vi "Bila-Sonatina.vi"(11 "NXT/EV3":T1) -> (3 "NXT/EV3 2":T1)   [LabVIEW 2016]
uses:
  <vilib>/NXT/Subs/LVHSConnector.ctl
  <vilib>/NXT/LegoClasses/BrickReference/BrickReference.lvclass
  <vilib>/NXT/Dual Mode Library/Display/drawText_Center.vi
  <vilib>/NXT/Dual Mode Library/Sound/PlayG.vi
  <vilib>/NXT/Dual Mode Library/Waits/Wait_Num.vi
  <vilib>/NXT/Dual Mode Library/Sound/PlayB.vi
  <vilib>/NXT/Dual Mode Library/Sound/PlayA.vi
  <vilib>/NXT/Dual Mode Library/Sound/PlayD.vi
  <vilib>/NXT/Dual Mode Library/Sound/PlayC.vi
  <vilib>/NXT/Dual Mode Library/Sound/PlayE.vi
  <vilib>/NXT/Dual Mode Library/Sound/PlayFsharp.vi
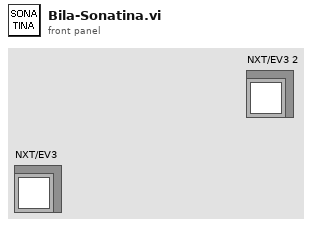
[diagram p1: front panel]
types:
  T1 = typedef "LVHSConnector.ctl" = refnum<class "BrickReference.lvclass">
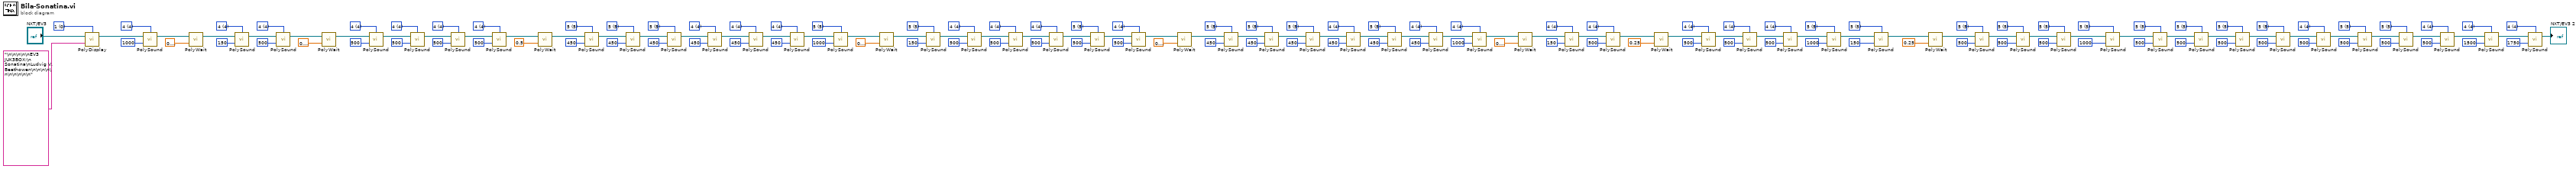
[diagram p0: block diagram]
diagram:
  w6 = u16 4 items=["3"=3, "4"=4, "5"=5, "6"=6, "7"=7] ("Octave")
  w10 = u16 5 items=["3"=3, "4"=4, "5"=5, "6"=6, "7"=7] ("Octave")
  w17 = u16 4 items=["3"=3, "4"=4, "5"=5, "6"=6, "7"=7] ("Octave")
  w20 = u16 4 items=["3"=3, "4"=4, "5"=5, "6"=6, "7"=7] ("Octave")
  w21 = u16 5 items=["3"=3, "4"=4, "5"=5, "6"=6, "7"=7] ("Octave")
  w24 = u16 4 items=["3"=3, "4"=4, "5"=5, "6"=6, "7"=7] ("Octave")
  w25 = u16 5 items=["3"=3, "4"=4, "5"=5, "6"=6, "7"=7] ("Octave")
  w28 = u16 5 items=["3"=3, "4"=4, "5"=5, "6"=6, "7"=7] ("Octave")
  w29 = u16 5 items=["3"=3, "4"=4, "5"=5, "6"=6, "7"=7] ("Octave")
  w32 = u16 5 items=["3"=3, "4"=4, "5"=5, "6"=6, "7"=7] ("Octave")
  w42 = u16 5 items=["3"=3, "4"=4, "5"=5, "6"=6, "7"=7] ("Octave")
  w41 = u16 5 items=["3"=3, "4"=4, "5"=5, "6"=6, "7"=7] ("Octave")
  w38 = u16 5 items=["3"=3, "4"=4, "5"=5, "6"=6, "7"=7] ("Octave")
  w37 = u16 5 items=["3"=3, "4"=4, "5"=5, "6"=6, "7"=7] ("Octave")
  w34 = u16 5 items=["3"=3, "4"=4, "5"=5, "6"=6, "7"=7] ("Octave")
  w62 = u16 5 items=["3"=3, "4"=4, "5"=5, "6"=6, "7"=7] ("Octave")
  w63 = u16 4 items=["3"=3, "4"=4, "5"=5, "6"=6, "7"=7] ("Octave")
  w66 = u16 4 items=["3"=3, "4"=4, "5"=5, "6"=6, "7"=7] ("Octave")
  w67 = u16 4 items=["3"=3, "4"=4, "5"=5, "6"=6, "7"=7] ("Octave")
  w70 = u16 4 items=["3"=3, "4"=4, "5"=5, "6"=6, "7"=7] ("Octave")
  w71 = u16 4 items=["3"=3, "4"=4, "5"=5, "6"=6, "7"=7] ("Octave")
  w74 = u16 4 items=["3"=3, "4"=4, "5"=5, "6"=6, "7"=7] ("Octave")
  w84 = u16 4 items=["3"=3, "4"=4, "5"=5, "6"=6, "7"=7] ("Octave")
  w85 = u16 5 items=["3"=3, "4"=4, "5"=5, "6"=6, "7"=7] ("Octave")
  w87 = u16 4 items=["3"=3, "4"=4, "5"=5, "6"=6, "7"=7] ("Octave")
  w90 = u16 5 items=["3"=3, "4"=4, "5"=5, "6"=6, "7"=7] ("Octave")
  w91 = u16 5 items=["3"=3, "4"=4, "5"=5, "6"=6, "7"=7] ("Octave")
  w94 = u16 5 items=["3"=3, "4"=4, "5"=5, "6"=6, "7"=7] ("Octave")
  w96 = u16 4 items=["3"=3, "4"=4, "5"=5, "6"=6, "7"=7] ("Octave")
  w111 = u16 5 items=["3"=3, "4"=4, "5"=5, "6"=6, "7"=7] ("Octave")
  w108 = u16 4 items=["3"=3, "4"=4, "5"=5, "6"=6, "7"=7] ("Octave")
  w107 = u16 4 items=["3"=3, "4"=4, "5"=5, "6"=6, "7"=7] ("Octave")
  w104 = u16 4 items=["3"=3, "4"=4, "5"=5, "6"=6, "7"=7] ("Octave")
  w103 = u16 5 items=["3"=3, "4"=4, "5"=5, "6"=6, "7"=7] ("Octave")
  w100 = u16 5 items=["3"=3, "4"=4, "5"=5, "6"=6, "7"=7] ("Octave")
  w124 = u16 4 items=["3"=3, "4"=4, "5"=5, "6"=6, "7"=7] ("Octave")
  w127 = u16 4 items=["3"=3, "4"=4, "5"=5, "6"=6, "7"=7] ("Octave")
  w131 = u16 4 items=["3"=3, "4"=4, "5"=5, "6"=6, "7"=7] ("Octave")
  w128 = u16 5 items=["3"=3, "4"=4, "5"=5, "6"=6, "7"=7] ("Octave")
  w134 = u16 5 items=["3"=3, "4"=4, "5"=5, "6"=6, "7"=7] ("Octave")
  w137 = u16 5 items=["3"=3, "4"=4, "5"=5, "6"=6, "7"=7] ("Octave")
  w150 = u16 4 items=["3"=3, "4"=4, "5"=5, "6"=6, "7"=7] ("Octave")
  w151 = u16 4 items=["3"=3, "4"=4, "5"=5, "6"=6, "7"=7] ("Octave")
  w154 = u16 4 items=["3"=3, "4"=4, "5"=5, "6"=6, "7"=7] ("Octave")
  w155 = u16 4 items=["3"=3, "4"=4, "5"=5, "6"=6, "7"=7] ("Octave")
  w158 = u16 4 items=["3"=3, "4"=4, "5"=5, "6"=6, "7"=7] ("Octave")
  w159 = u16 4 items=["3"=3, "4"=4, "5"=5, "6"=6, "7"=7] ("Octave")
  w162 = u16 4 items=["3"=3, "4"=4, "5"=5, "6"=6, "7"=7] ("Octave")
  w164 = i16 0 items=["1", "2", "3", "4", "5", "6", "7", "8", "9", "10", "11", "12"] ("Line")
  n1 = call-poly <vilib>:"PolyDisplay.vi"("Text"="\n\n\n\n\nEV3 JUK3BOX:\n Sonatina\nLudvig V. Beethowen\n\n\n\n\n\n\n\n\n\n", "NXT/EV3"="NXT/EV3", "Line"=w164) -> ("NXT/EV3"=w144:T1)  [unwired: 1 in]
  n2 = call-poly <vilib>:"PolySound.vi"("Duration (500 ms)"=u16 1000, "NXT/EV3"=w144, "Octave"=w162) -> ("NXT/EV3"=w141:T1)  [unwired: 1 in]
  n3 = call-poly <vilib>:"PolyWait.vi"("Time (1 sec)"=sgl 0.1, "NXT/EV3"=w141) -> ("NXT/EV3"=w142:T1)  [unwired: 2 in]
  n4 = call-poly <vilib>:"PolySound.vi"("Duration (500 ms)"=u16 150, "NXT/EV3"=w142, "Octave"=w159) -> ("NXT/EV3"=w148:T1)  [unwired: 1 in]
  n5 = call-poly <vilib>:"PolySound.vi"("Duration (500 ms)"=u16 500, "NXT/EV3"=w148, "Octave"=w158) -> ("NXT/EV3"=w139:T1)  [unwired: 1 in]
  n6 = call-poly <vilib>:"PolyWait.vi"("Time (1 sec)"=sgl 0.1, "NXT/EV3"=w139) -> ("NXT/EV3"=w138:T1)  [unwired: 2 in]
  n7 = call-poly <vilib>:"PolySound.vi"("Duration (500 ms)"=u16 500, "NXT/EV3"=w138, "Octave"=w155) -> ("NXT/EV3"=w147:T1)  [unwired: 1 in]
  n8 = call-poly <vilib>:"PolySound.vi"("Duration (500 ms)"=u16 500, "NXT/EV3"=w147, "Octave"=w154) -> ("NXT/EV3"=w146:T1)  [unwired: 1 in]
  n9 = call-poly <vilib>:"PolySound.vi"("Duration (500 ms)"=u16 500, "NXT/EV3"=w146, "Octave"=w151) -> ("NXT/EV3"=w145:T1)  [unwired: 1 in]
  n10 = call-poly <vilib>:"PolySound.vi"("Duration (500 ms)"=u16 500, "NXT/EV3"=w145, "Octave"=w150) -> ("NXT/EV3"=w119:T1)  [unwired: 1 in]
  n11 = call-poly <vilib>:"PolyWait.vi"("Time (1 sec)"=sgl 0.5, "NXT/EV3"=w119) -> ("NXT/EV3"=w120:T1)  [unwired: 2 in]
  n12 = call-poly <vilib>:"PolySound.vi"("Duration (500 ms)"=u16 450, "NXT/EV3"=w120, "Octave"=w137) -> ("NXT/EV3"=w133:T1)  [unwired: 1 in]
  n13 = call-poly <vilib>:"PolySound.vi"("Duration (500 ms)"=u16 450, "NXT/EV3"=w133, "Octave"=w134) -> ("NXT/EV3"=w122:T1)  [unwired: 1 in]
  n14 = call-poly <vilib>:"PolySound.vi"("Duration (500 ms)"=u16 450, "NXT/EV3"=w122, "Octave"=w128) -> ("NXT/EV3"=w132:T1)  [unwired: 1 in]
  n15 = call-poly <vilib>:"PolySound.vi"("Duration (500 ms)"=u16 450, "NXT/EV3"=w132, "Octave"=w131) -> ("NXT/EV3"=w121:T1)  [unwired: 1 in]
  n16 = call-poly <vilib>:"PolySound.vi"("Duration (500 ms)"=u16 450, "NXT/EV3"=w121, "Octave"=w127) -> ("NXT/EV3"=w123:T1)  [unwired: 1 in]
  n17 = call-poly <vilib>:"PolySound.vi"("Duration (500 ms)"=u16 450, "NXT/EV3"=w123, "Octave"=w124) -> ("NXT/EV3"=w99:T1)  [unwired: 1 in]
  n18 = call-poly <vilib>:"PolySound.vi"("Duration (500 ms)"=u16 1000, "NXT/EV3"=w99, "Octave"=w100) -> ("NXT/EV3"=w117:T1)  [unwired: 1 in]
  n19 = call-poly <vilib>:"PolyWait.vi"("Time (1 sec)"=sgl 0.1, "NXT/EV3"=w117) -> ("NXT/EV3"=w116:T1)  [unwired: 2 in]
  n20 = call-poly <vilib>:"PolySound.vi"("Duration (500 ms)"=u16 150, "NXT/EV3"=w116, "Octave"=w103) -> ("NXT/EV3"=w112:T1)  [unwired: 1 in]
  n21 = call-poly <vilib>:"PolySound.vi"("Duration (500 ms)"=u16 500, "NXT/EV3"=w112, "Octave"=w104) -> ("NXT/EV3"=w98:T1)  [unwired: 1 in]
  n22 = call-poly <vilib>:"PolySound.vi"("Duration (500 ms)"=u16 500, "NXT/EV3"=w98, "Octave"=w107) -> ("NXT/EV3"=w113:T1)  [unwired: 1 in]
  n23 = call-poly <vilib>:"PolySound.vi"("Duration (500 ms)"=u16 500, "NXT/EV3"=w113, "Octave"=w108) -> ("NXT/EV3"=w114:T1)  [unwired: 1 in]
  n24 = call-poly <vilib>:"PolySound.vi"("Duration (500 ms)"=u16 500, "NXT/EV3"=w114, "Octave"=w111) -> ("NXT/EV3"=w95:T1)  [unwired: 1 in]
  n25 = call-poly <vilib>:"PolySound.vi"("Duration (500 ms)"=u16 500, "NXT/EV3"=w95, "Octave"=w96) -> ("NXT/EV3"=w77:T1)  [unwired: 1 in]
  n26 = call-poly <vilib>:"PolyWait.vi"("Time (1 sec)"=sgl 0.1, "NXT/EV3"=w77) -> ("NXT/EV3"=w76:T1)  [unwired: 2 in]
  n27 = call-poly <vilib>:"PolySound.vi"("Duration (500 ms)"=u16 450, "NXT/EV3"=w76, "Octave"=w94) -> ("NXT/EV3"=w82:T1)  [unwired: 1 in]
  n28 = call-poly <vilib>:"PolySound.vi"("Duration (500 ms)"=u16 450, "NXT/EV3"=w82, "Octave"=w91) -> ("NXT/EV3"=w81:T1)  [unwired: 1 in]
  n29 = call-poly <vilib>:"PolySound.vi"("Duration (500 ms)"=u16 450, "NXT/EV3"=w81, "Octave"=w90) -> ("NXT/EV3"=w80:T1)  [unwired: 1 in]
  n30 = call-poly <vilib>:"PolySound.vi"("Duration (500 ms)"=u16 450, "NXT/EV3"=w80, "Octave"=w87) -> ("NXT/EV3"=w75:T1)  [unwired: 1 in]
  n31 = call-poly <vilib>:"PolySound.vi"("Duration (500 ms)"=u16 450, "NXT/EV3"=w75, "Octave"=w85) -> ("NXT/EV3"=w79:T1)  [unwired: 1 in]
  n32 = call-poly <vilib>:"PolySound.vi"("Duration (500 ms)"=u16 450, "NXT/EV3"=w79, "Octave"=w84) -> ("NXT/EV3"=w51:T1)  [unwired: 1 in]
  n33 = call-poly <vilib>:"PolySound.vi"("Duration (500 ms)"=u16 1000, "NXT/EV3"=w51, "Octave"=w74) -> ("NXT/EV3"=w55:T1)  [unwired: 1 in]
  n34 = call-poly <vilib>:"PolyWait.vi"("Time (1 sec)"=sgl 0.1, "NXT/EV3"=w55) -> ("NXT/EV3"=w56:T1)  [unwired: 2 in]
  n35 = call-poly <vilib>:"PolySound.vi"("Duration (500 ms)"=u16 150, "NXT/EV3"=w56, "Octave"=w71) -> ("NXT/EV3"=w60:T1)  [unwired: 1 in]
  n36 = call-poly <vilib>:"PolySound.vi"("Duration (500 ms)"=u16 500, "NXT/EV3"=w60, "Octave"=w70) -> ("NXT/EV3"=w53:T1)  [unwired: 1 in]
  n37 = call-poly <vilib>:"PolyWait.vi"("Time (1 sec)"=sgl 0.25, "NXT/EV3"=w53) -> ("NXT/EV3"=w52:T1)  [unwired: 2 in]
  n38 = call-poly <vilib>:"PolySound.vi"("Duration (500 ms)"=u16 500, "NXT/EV3"=w52, "Octave"=w67) -> ("NXT/EV3"=w59:T1)  [unwired: 1 in]
  n39 = call-poly <vilib>:"PolySound.vi"("Duration (500 ms)"=u16 500, "NXT/EV3"=w59, "Octave"=w66) -> ("NXT/EV3"=w58:T1)  [unwired: 1 in]
  n40 = call-poly <vilib>:"PolySound.vi"("Duration (500 ms)"=u16 500, "NXT/EV3"=w58, "Octave"=w63) -> ("NXT/EV3"=w50:T1)  [unwired: 1 in]
  n41 = call-poly <vilib>:"PolySound.vi"("Duration (500 ms)"=u16 1000, "NXT/EV3"=w50, "Octave"=w62) -> ("NXT/EV3"=w33:T1)  [unwired: 1 in]
  n42 = call-poly <vilib>:"PolySound.vi"("Duration (500 ms)"=u16 150, "NXT/EV3"=w33, "Octave"=w34) -> ("NXT/EV3"=w47:T1)  [unwired: 1 in]
  n43 = call-poly <vilib>:"PolyWait.vi"("Time (1 sec)"=sgl 0.25, "NXT/EV3"=w47) -> ("NXT/EV3"=w48:T1)  [unwired: 2 in]
  n44 = call-poly <vilib>:"PolySound.vi"("Duration (500 ms)"=u16 500, "NXT/EV3"=w48, "Octave"=w37) -> ("NXT/EV3"=w44:T1)  [unwired: 1 in]
  n45 = call-poly <vilib>:"PolySound.vi"("Duration (500 ms)"=u16 500, "NXT/EV3"=w44, "Octave"=w38) -> ("NXT/EV3"=w45:T1)  [unwired: 1 in]
  n46 = call-poly <vilib>:"PolySound.vi"("Duration (500 ms)"=u16 500, "NXT/EV3"=w45, "Octave"=w41) -> ("NXT/EV3"=w49:T1)  [unwired: 1 in]
  n47 = call-poly <vilib>:"PolySound.vi"("Duration (500 ms)"=u16 1000, "NXT/EV3"=w49, "Octave"=w42) -> ("NXT/EV3"=w3:T1)  [unwired: 1 in]
  n48 = call-poly <vilib>:"PolySound.vi"("Duration (500 ms)"=u16 500, "NXT/EV3"=w3, "Octave"=w32) -> ("NXT/EV3"=w16:T1)  [unwired: 1 in]
  n49 = call-poly <vilib>:"PolySound.vi"("Duration (500 ms)"=u16 500, "NXT/EV3"=w16, "Octave"=w29) -> ("NXT/EV3"=w15:T1)  [unwired: 1 in]
  n50 = call-poly <vilib>:"PolySound.vi"("Duration (500 ms)"=u16 500, "NXT/EV3"=w15, "Octave"=w28) -> ("NXT/EV3"=w14:T1)  [unwired: 1 in]
  n51 = call-poly <vilib>:"PolySound.vi"("Duration (500 ms)"=u16 500, "NXT/EV3"=w14, "Octave"=w25) -> ("NXT/EV3"=w13:T1)  [unwired: 1 in]
  n52 = call-poly <vilib>:"PolySound.vi"("Duration (500 ms)"=u16 500, "NXT/EV3"=w13, "Octave"=w24) -> ("NXT/EV3"=w12:T1)  [unwired: 1 in]
  n53 = call-poly <vilib>:"PolySound.vi"("Duration (500 ms)"=u16 500, "NXT/EV3"=w12, "Octave"=w21) -> ("NXT/EV3"=w8:T1)  [unwired: 1 in]
  n54 = call-poly <vilib>:"PolySound.vi"("Duration (500 ms)"=u16 500, "NXT/EV3"=w8, "Octave"=w10) -> ("NXT/EV3"=w7:T1)  [unwired: 1 in]
  n55 = call-poly <vilib>:"PolySound.vi"("Duration (500 ms)"=u16 500, "NXT/EV3"=w7, "Octave"=w20) -> ("NXT/EV3"=w11:T1)  [unwired: 1 in]
  n56 = call-poly <vilib>:"PolySound.vi"("Duration (500 ms)"=u16 1500, "NXT/EV3"=w11, "Octave"=w17) -> ("NXT/EV3"=w4:T1)  [unwired: 1 in]
  n57 = call-poly <vilib>:"PolySound.vi"("Duration (500 ms)"=u16 1750, "NXT/EV3"=w4, "Octave"=w6) -> ("NXT/EV3"=→"NXT/EV3 2":T1)  [unwired: 1 in]
